vi "Get Cell (String).vi"(6 "Column":i32, 8 "error in (no error)":errorcluster, 9 "Row":i32, 10 "Sheet Reference":refnum<k24>) -> (0 "error out":errorcluster, 2 "Sheet Reference out":refnum<k24>, 5 "Value":string)   [LabVIEW 2014]
uses:
  C:/Users/LENOVO/Desktop/CodeSpace GUI/LVExcel/Resources/net40/NPOI.dll
  Resources/net40/NPOI.dll
  <vilib>/ErrorRing/Error Ring.xnode
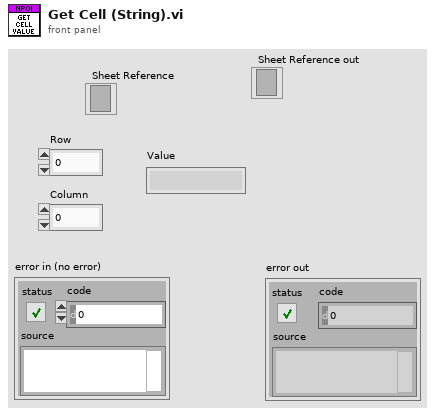
[diagram p1: front panel]
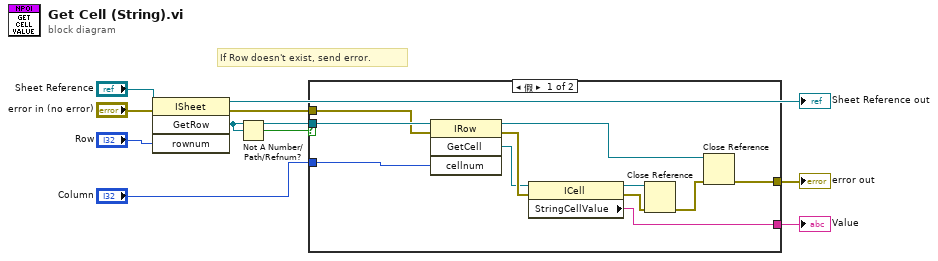
[diagram p0: block diagram]
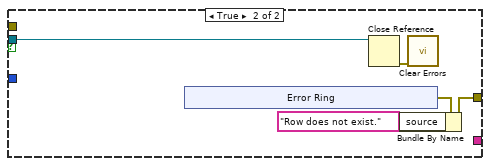
[diagram p2: hidden frame]
diagram:
  # "If Row doesn't exist, send error."
  n1 = invoke class="ISheet" method="GetRow"(reference="Sheet Reference", error in="error in (no error)", "rownum"="Row") -> (reference out=→"Sheet Reference out":refnum<k24>, error out=w3:errorcluster, "GetRow"=w8:refnum<k24>)  [unwired: 1 in, 1 out]
  n2 = Not A Number/Path/Refnum?(number/path/refnum=w8) -> (NaN/Path/Refnum?=w2:bool)
  n3 = case shown="假" w2 {
    tunnel: "Column" -> [w20 _]
    tunnel: [w18 w23] -> w9
    tunnel: w8 -> [w17 w26]
    tunnel: w3 -> [w16 _]
    tunnel: [w11 _] -> w1
    frame False {
      n4 = invoke class="IRow" method="GetCell"(reference=w17, error in=w16, "cellnum"=w20) -> (reference out=w21:refnum<k24>, error out=w15:errorcluster, "GetCell"=w14:refnum<k24>)  [unwired: 1 in, 1 out]
      n5 = property class="ICell"(reference=w14, error in=w15) -> (reference out=w12:refnum<k24>, error out=w13:errorcluster, "StringCellValue"=w11:string)
      n6 = Close Reference(reference=w12, error in (no error)=w13) -> (error out=w19:errorcluster)
      n7 = Close Reference(reference=w21, error in (no error)=w19) -> (error out=w18:errorcluster)
    }
    frame True {
      n8 = xnode "Error Ring"() -> ("错误输出"=w24:errorcluster)
      n9 = Close Reference(reference=w26) -> (error out=w25:errorcluster)  [unwired: 1 in]
      n10 = Bundle By Name(cluster=w24, "source"="Row does not exist.") -> (w23:errorcluster)
      n11 = call <vilib>:"Clear Errors.vi"("error in (no error)"=w25) -> ()  [unwired: 5 in, 2 out]
    }
  }
  "error out" <- w9
  "Value" <- w1
